vi "Parse and Log Event Data.vi"(8 "error in (no error)":errorcluster, 10 "Event Variant":variant, 11 "Report Generator in":refnum<class "Report Generator.lvclass">) -> (0 "error out":errorcluster, 3 "Report Generator out":refnum<class "Report Generator.lvclass">)   [LabVIEW 2023, in "Report Generator.lvlib" / "Report Generator.lvclass"]
doc: "This receives the event data variant, formats it to a cluster with:\n<b>Timestamp</b>\n<b>Source</b>\n<b>Event Description</b>\n<b>Event Details</b>"
uses:
  Library/Report Generator.lvclass
  Custom Controls/Event Data.ctl
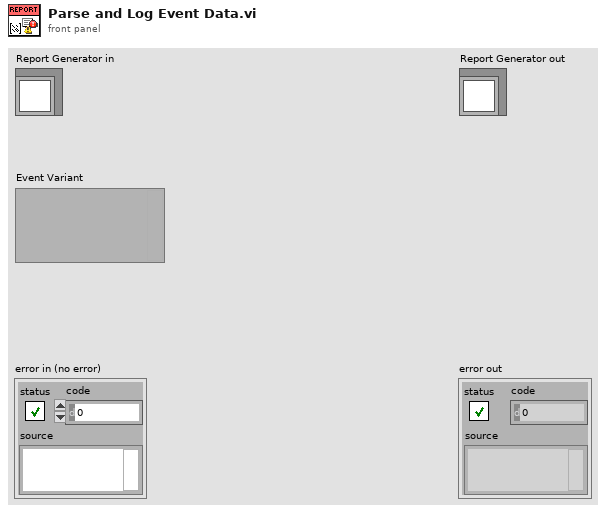
[diagram p1: front panel]
types:
  T1 = typedef "Report Generator.lvlib/Report Generator.lvclass/Event Data.ctl" = cluster{"Time Stamp":timestamp, "Source":string, "Description":string, "Details":string}
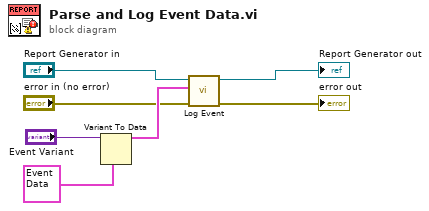
[diagram p0: block diagram]
diagram:
  n1 = Variant To Data(type=T1 {"Time Stamp"=timestamp(0 s since 1904-01-01), "Source"="", "Description"="", "Details"=""} ("Event Data"), Variant="Event Variant") -> (data=w3:T1)  [unwired: 1 in, 1 out]
  n2 = call-dynamic "Log Event.vi"("error in (no error)"="error in (no error)", "Event Data"=w3, "Report Generator in"="Report Generator in") -> ("error out"=→"error out":errorcluster, "Report Generator out"=→"Report Generator out":refnum<class "Report Generator.lvclass">)  [unwired: 7 in]
